vi "TicTacToev2.vi"() -> ()   [LabVIEW 2020]
panel:
  in  "Numeric":i32
  out "Who's Tern ?":bool
  out "Tank 2":i32(slide)
  out "players":dbl format="%#g"
  in  "LEVEL":i32(slide)=3000 scale=5.0..1.0
  out "Tank":i32(slide)
  out "Human(GREEN) Win":dbl
  out "Computer(RED)Win":dbl
  out "Tie":bool
  out "No one Won":bool
  out "Computer Won":bool
  out "Human Won":bool
  out "Turn":string
  out "XO array":string[][](array[string])
  in  "START GAME":bool
  in  "Boolean 9":bool
  in  "Boolean 8":bool
  in  "Boolean 7":bool
  in  "Boolean 6":bool
  in  "Boolean 5":bool
  in  "Boolean 4":bool
  in  "Boolean 3":bool
  in  "Boolean 2":bool
  in  "Boolean":bool
  in  "STOP GAME":bool
  in  "Turn":bool
  out "Game Over":bool
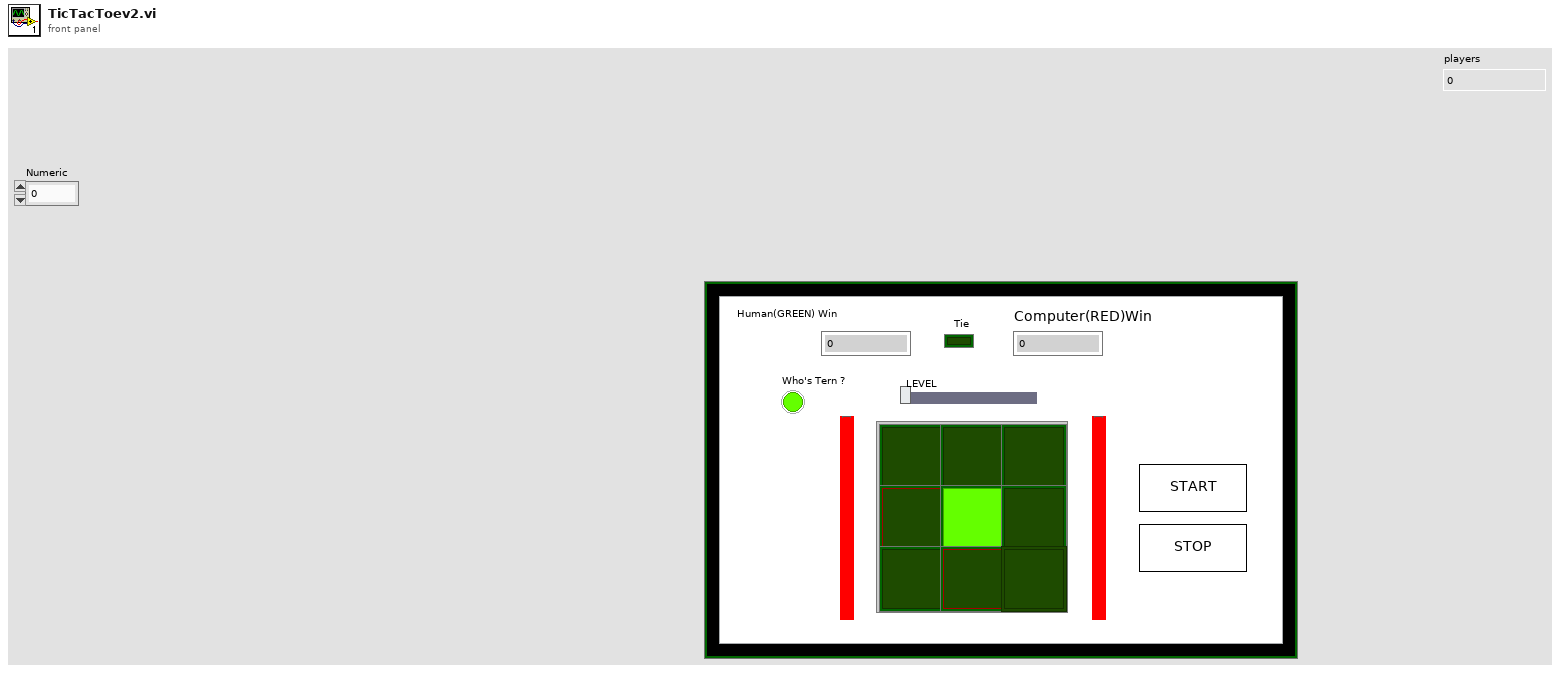
[diagram p1: front panel]
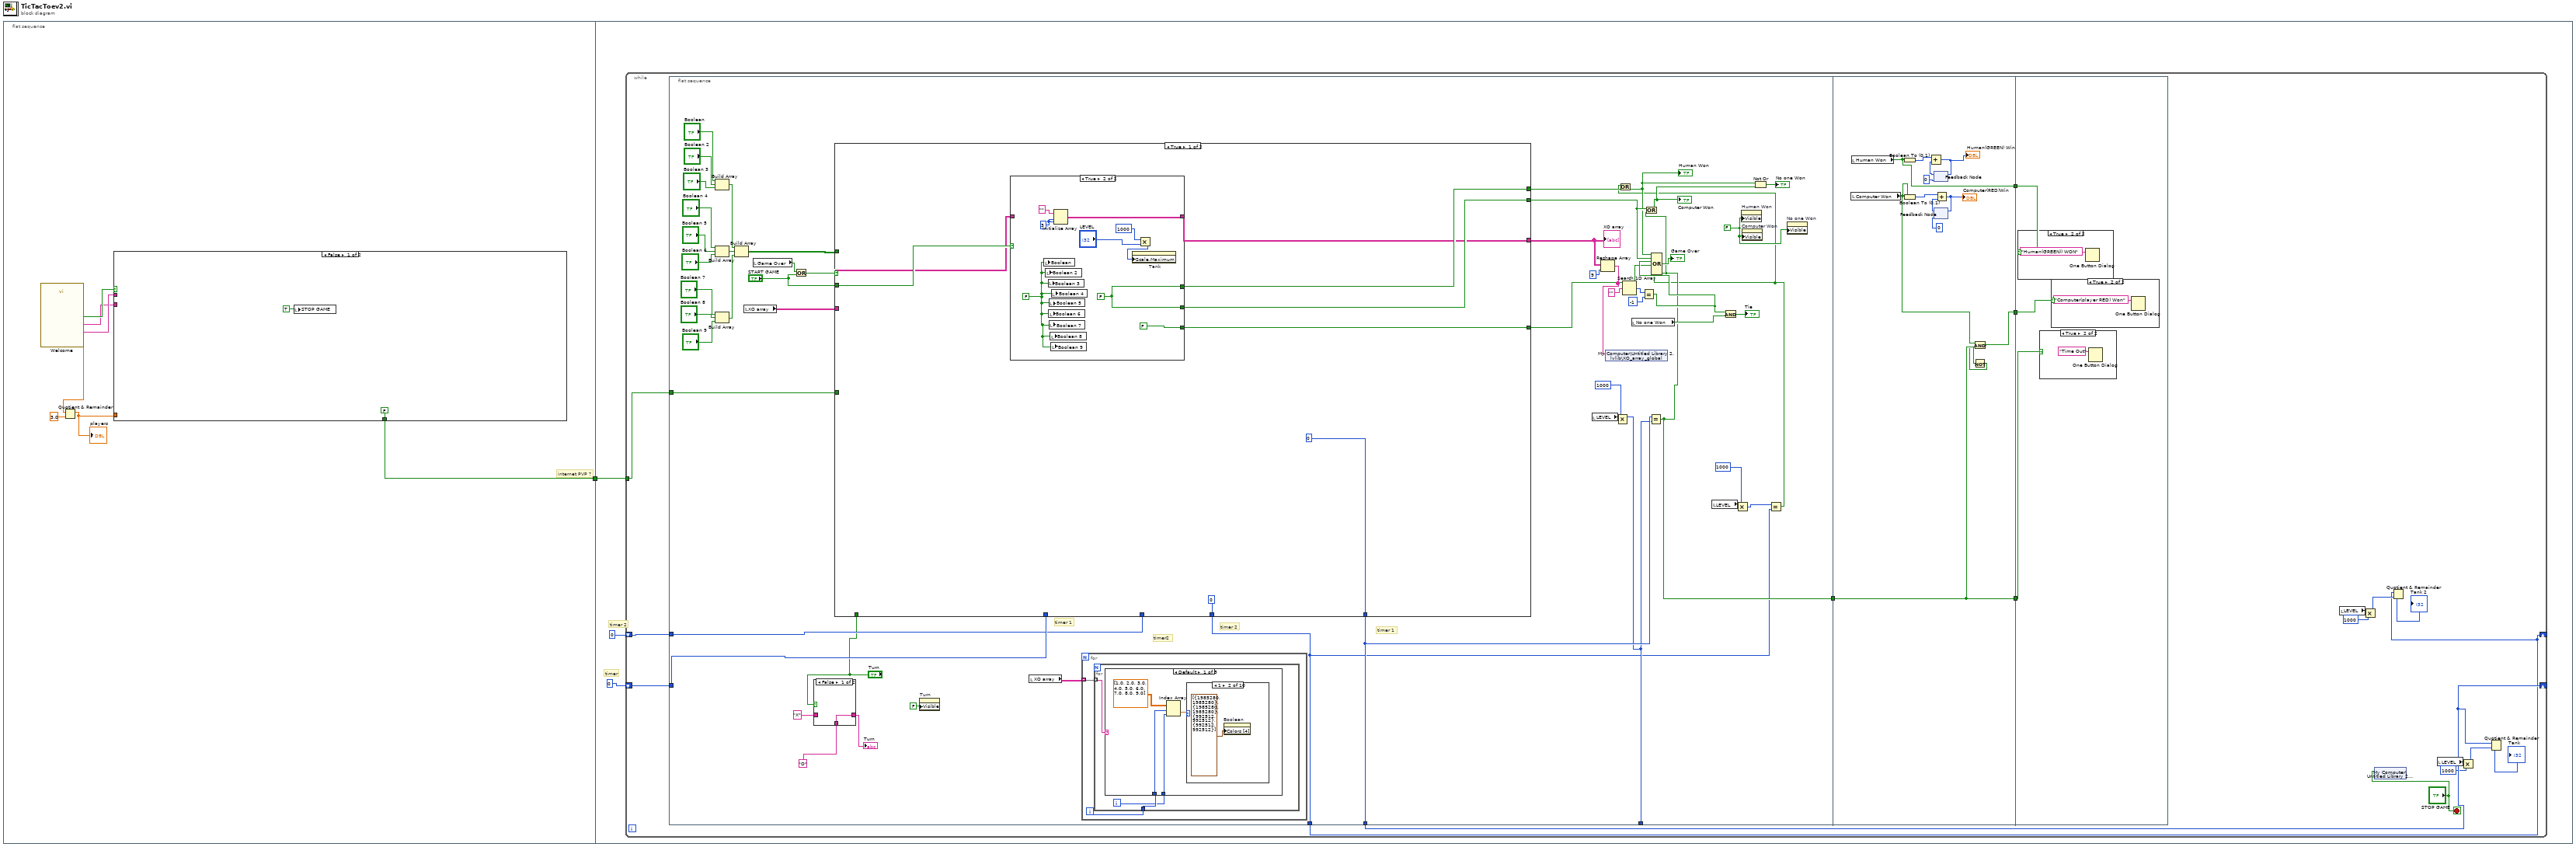
[diagram p0: block diagram]
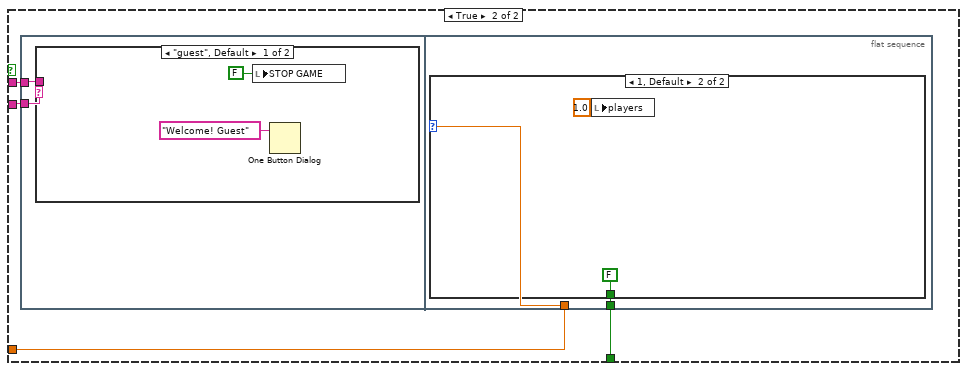
[diagram p2: hidden frame]
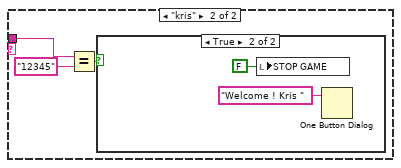
[diagram p3: hidden frame]
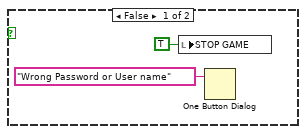
[diagram p4: hidden frame]
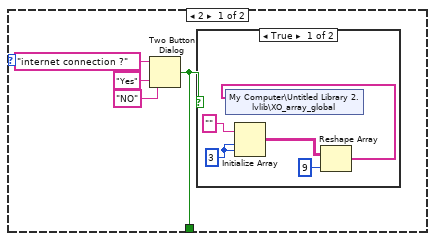
[diagram p5: hidden frame]
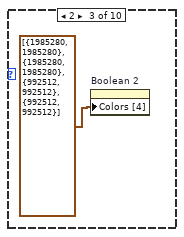
[diagram p8: hidden frame]
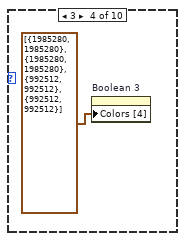
[diagram p9: hidden frame]
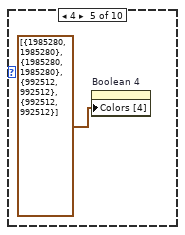
[diagram p10: hidden frame]
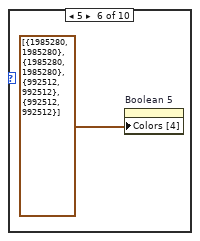
[diagram p11: hidden frame]
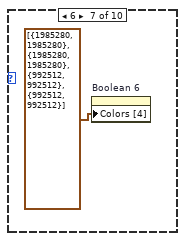
[diagram p12: hidden frame]
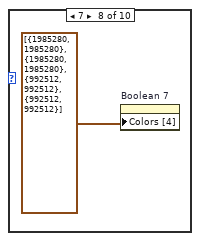
[diagram p13: hidden frame]
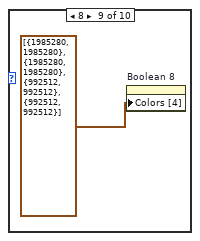
[diagram p14: hidden frame]
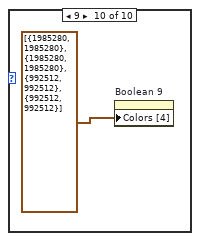
[diagram p15: hidden frame]
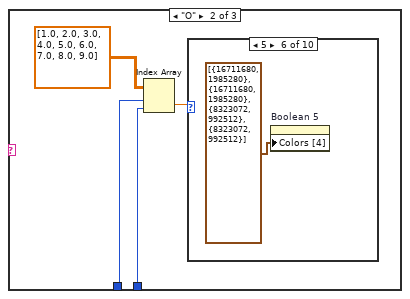
[diagram p16: hidden frame]
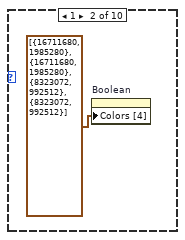
[diagram p18: hidden frame]
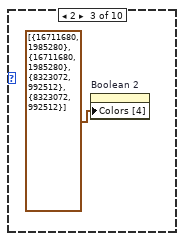
[diagram p19: hidden frame]
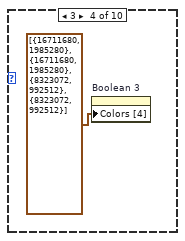
[diagram p20: hidden frame]
diagram:
  n1 = flat-sequence {
    tunnel: [w2] -> w1
    tunnel: w1 -> [w39]
    frame #0 {
      # "internet PVP ?"
      n2 = call "Welcome"() -> ("players(1 or 2 )"=w8:dbl, "password"=w5:string, "name"=w4:string, "OK"=w7:bool)  [unwired: 15 in, 1 out]
      n3 = Quotient & Remainder(x=w8, y=3.0) -> (x-y*floor(x/y)=w3:dbl)  [unwired: 1 out]
      "players" <- w3
      n4 = case shown="False" w7 {
        tunnel: w4 -> [_ w14]
        tunnel: w5 -> [_ w13]
        tunnel: w3 -> [_ w12]
        tunnel: [FALSE ("T button?") w11] -> w2
        frame False {
          n5 = local write "STOP GAME"(TRUE ("STOP GAME")) -> ()
        }
        frame True {
          n6 = flat-sequence {
            tunnel: w14 -> [w16]
            tunnel: w13 -> [w15]
            tunnel: w12 -> [w27]
            tunnel: [w26] -> w11
            frame #0 {
              n7 = case shown="\"guest\", Default" w16 {
                tunnel: w15 -> [_ w21]
                frame "guest", Default {
                  n8 = local write "STOP GAME"(FALSE ("STOP GAME")) -> ()
                  n9 = One Button Dialog(message="Welcome! Guest") -> ()  [unwired: 1 in, 1 out]
                }
                frame "kris" {
                  n10 = Equal?(x=w21, y="12345") -> (x = y?=w19:bool)
                  n11 = case shown="True" w19 {
                    frame False {
                      n12 = local write "STOP GAME"(TRUE ("STOP GAME")) -> ()
                      n13 = One Button Dialog(message="Wrong Password or User name") -> ()  [unwired: 1 in, 1 out]
                    }
                    frame True {
                      n14 = local write "STOP GAME"(FALSE ("STOP GAME")) -> ()
                      n15 = One Button Dialog(message="Welcome ! Kris ") -> ()  [unwired: 1 in, 1 out]
                    }
                  }
                }
              }
            }
            frame #1 {
              n16 = case shown="1, Default" w27 {
                tunnel: [w28 FALSE ("T button?")] -> w26
                frame 2 {
                  n17 = Two Button Dialog(message="internet connection ?", 1:"NO" ("F button name (\"Cancel\")"), 2:"Yes" ("T button name (\"OK\")")) -> (T button?=w28:bool)
                  n18 = case shown="True" w28 {
                    frame True {
                      w36 = 3
                      n19 = Initialize Array("", w36, w36) -> (w33:string[][])
                      n20 = Reshape Array(w33, 9 ("dimension size")) -> (w32:string[])
                      n21 = shared-variable "My Computer\\Untitled Library 2.lvlib\\XO_array_global"(w32) -> ()  [unwired: 1 in, 1 out]
                    }
                    frame False {
                    }
                  }
                }
                frame 1, Default {
                  n22 = local write "players"(1.0 ("players")) -> ()
                }
              }
            }
          }
        }
      }
    }
    frame #1 {
      # "timer 2"
      # "timer"
      n23 = while {
        shift-right: [w55] -> _
        shift-left: 0 -> [w57]
        shift-right: [w44] -> _
        shift-left: 0 -> [w49]
        tunnel: w39 -> [w42]
        stop <- "STOP GAME" stop-if-true
        n24 = flat-sequence {
          tunnel: [w75] -> w55
          tunnel: [w73] -> w53
          tunnel: [w71] -> _
          tunnel: w57 -> [w76]
          tunnel: w49 -> [w69]
          tunnel: [w65] -> w44
          tunnel: w42 -> [w61]
          tunnel: [w316] -> w59
          tunnel: [w319] -> w58
          tunnel: [w318] -> w54
          tunnel: w53 -> [w318]
          tunnel: w59 -> [w330]
          tunnel: w58 -> [w329]
          tunnel: w54 -> [w328]
          frame #0 {
            w78 = FALSE ("Visible")
            # "timer 1"
            # "timer 2"
            # "timer 1"
            # "timer2"
            n25 = Build Array("Boolean", "Boolean 2", "Boolean 3") -> (w110:bool[])
            n26 = Build Array("Boolean 4", "Boolean 5", "Boolean 6") -> (w111:bool[])
            n27 = Build Array("Boolean 7", "Boolean 8", "Boolean 9") -> (w112:bool[])
            n28 = Build Array(w110, w111, w112) -> (w102:bool[][])
            n29 = local read "XO array"() -> (w101:string[][])
            n30 = local read "Game Over"() -> (w94:bool)
            n31 = Or(x=w94, y="START GAME") -> (x .or. y?=w93:bool)
            n32 = case shown="False" "Turn" {
              tunnel: "X" -> [_ w158]
              tunnel: [w157 w158] -> w99
              tunnel: "O" ("x") -> [w157 _]
              frame False {
              }
              frame True {
              }
            }
            "Turn" <- w99
            n33 = case shown="True" w93 {
              tunnel: w102 -> [_ w200]
              tunnel: w101 -> [w165 w199]
              tunnel: "Turn" -> [_ w198]
              tunnel: "START GAME" -> [w166 _]
              tunnel: [w164 w191] -> w80
              tunnel: [w163 w190] -> w79
              tunnel: [w162 w189] -> w83
              tunnel: [w161 FALSE] -> w77
              tunnel: w76 -> [_ w187]
              tunnel: [0 w186] -> w75
              tunnel: w69 -> [_ w185]
              tunnel: [0 w184] -> w65
              tunnel: w61 -> [_ w180]
              frame True {
                n34 = case shown="True" w166 {
                  tunnel: [w169 w177] -> w162
                  tunnel: [w168 w176] -> w163
                  tunnel: [w168 w176] -> w164
                  tunnel: w165 -> [w169 _]
                  tunnel: [TRUE FALSE] -> w161
                  frame False {
                    w168 = FALSE
                  }
                  frame True {
                    w174 = FALSE
                    w176 = FALSE
                    w175 = 3
                    n35 = local write "Boolean"(w174) -> ()
                    n36 = local write "Boolean 2"(w174) -> ()
                    n37 = local write "Boolean 3"(w174) -> ()
                    n38 = local write "Boolean 6"(w174) -> ()
                    n39 = local write "Boolean 5"(w174) -> ()
                    n40 = local write "Boolean 7"(w174) -> ()
                    n41 = local write "Boolean 8"(w174) -> ()
                    n42 = local write "Boolean 9"(w174) -> ()
                    n43 = local write "Boolean 4"(w174) -> ()
                    n44 = Initialize Array("", w175, w175) -> (w177:string[][])
                    n45 = Multiply(x=1000, y="LEVEL") -> (x*y=w170:i32)
                    n46 = property on="Tank" class="Slide (strict)"("Scale.Maximum"=w170) -> ()  [unwired: 2 in, 2 out]
                  }
                }
              }
              frame False {
                n47 = local read "Turn"() -> (w179:string)
                n48 = shared-variable "My Computer\\Untitled Library 2.lvlib\\Turn_string"(w179) -> ()  [unwired: 1 in, 1 out]
                n49 = Equal?(x=w179, y="O") -> (x = y?=w182:bool)
                n50 = case shown="False" w182 {
                  frame False {
                    n51 = property on="Who's Tern ?" class="Bool (strict)"("Colors [4]"=cluster{u32, u32}[] [{6618880, 6618880}]) -> ()  [unwired: 2 in, 2 out]
                  }
                  frame True {
                    n52 = property on="Who's Tern ?" class="Bool (strict)"("Colors [4]"=cluster{u32, u32}[] [{16711680, 16711680}]) -> ()  [unwired: 2 in, 2 out]
                  }
                }
                n53 = case shown="False" w198 {
                  tunnel: w200 -> [w213 w285]
                  tunnel: w199 -> [w215 w284]
                  tunnel: [w216 w283] -> w189
                  tunnel: w179 -> [w212 w282]
                  tunnel: w187 -> [w208 w280]
                  tunnel: [w211 w279] -> w186
                  tunnel: w185 -> [w210 _]
                  tunnel: [w209 0] -> w184
                  tunnel: w180 -> [w207 _]
                  frame False {
                    n54 = local read "players"() -> (w214:dbl)
                    n55 = case shown="2" w214 {
                      tunnel: [w221 w276] -> w216
                      tunnel: w215 -> [w224 w275]
                      tunnel: w213 -> [w222 _]
                      tunnel: w212 -> [w223 _]
                      tunnel: w210 -> [w220 _]
                      tunnel: [0 0] -> w211
                      tunnel: [w219 0] -> w209
                      tunnel: w208 -> [_ _]
                      tunnel: w207 -> [w217 _]
                      frame 2 {
                        # "connect to timer2"
                        n56 = case shown="True" w217 {
                          tunnel: w224 -> [_ w240]
                          tunnel: w223 -> [_ w239]
                          tunnel: w222 -> [_ w238]
                          tunnel: [w226 w237] -> w221
                          tunnel: w220 -> [_ w236]
                          tunnel: ["Numeric" w235] -> w219
                          frame True {
                            n57 = flat-sequence {
                              tunnel: [w233] -> w226
                              frame #0 {
                                n58 = while {
                                stop <- w229 stop-if-true
                                n59 = shared-variable "My Computer\\Untitled Library 2.lvlib\\Internet_PVP"(TRUE ("Internet_PVP")) -> ()  [unwired: 1 in, 1 out]
                                n60 = shared-variable "My Computer\\Untitled Library 2.lvlib\\Turn"(FALSE ("Turn")) -> ()  [unwired: 1 in, 1 out]
                                n61 = shared-variable "My Computer\\Untitled Library 2.lvlib\\Client_end"() -> (w229:bool)  [unwired: 1 in, 1 out]
                                n62 = shared-variable "My Computer\\Untitled Library 2.lvlib\\timer_2"() -> (w228:i32)  [unwired: 1 in, 1 out]
                                n63 = local write "Numeric"(w228) -> ()
                                }
                              }
                              frame #1 {
                                n64 = shared-variable "My Computer\\Untitled Library 2.lvlib\\XO_array_global"() -> (w234:string[])  [unwired: 1 in, 1 out]
                                n65 = Reshape Array(w234, 3 ("dimension size"), 3 ("dimension size")) -> (w233:string[][])
                              }
                            }
                          }
                          frame False {
                            w241 = 3
                            n66 = for {
                              N: w241 -> [_]
                              tunnel: w241 -> [w248]
                              tunnel: w238 -> [w247] mode=indexing
                              tunnel: w240 -> [w246] mode=indexing
                              tunnel: [w245] -> w237 mode=indexing
                              tunnel: w239 -> [w244]
                              tunnel: w236 -> [w243]
                              tunnel: [w242] -> w235
                              n67 = for {
                                N: w248 -> [_]
                                tunnel: w247 -> [w258] mode=indexing
                                tunnel: w246 -> [w255] mode=indexing
                                tunnel: w244 -> [w253]
                                tunnel: [w254] -> w245 mode=indexing
                                tunnel: w243 -> [w250]
                                tunnel: [w249] -> w242
                                n68 = Not Equal?(x=w255, y="X") -> (x != y?=w259:bool)
                                n69 = Not Equal?(x="O", y=w255) -> (x != y?=w260:bool)
                                n70 = And(x=w260, y=w259) -> (x .and. y?=w257:bool)
                                n71 = local read "Turn"() -> (w252:bool)
                                n72 = And(x=w258, y=w257) -> (x .and. y?=w256:bool)
                                n73 = case shown="True" w256 {
                                tunnel: w255 -> [w266 _]
                                tunnel: [w266 w268] -> w254
                                tunnel: w253 -> [_ w268]
                                tunnel: [w265 w269] -> w251
                                tunnel: w252 -> [w265 w270]
                                tunnel: w250 -> [w264 _]
                                tunnel: [w263 0] -> w249
                                frame False {
                                n74 = Increment(x=w264) -> (x+1=w263:i32)
                                }
                                frame True {
                                n75 = Not(x=w270) -> (.not. x?=w269:bool)
                                }
                                }
                                n76 = local write "Turn"(w251) -> ()
                              }
                            }
                          }
                        }
                      }
                      frame 1, Default {
                        n77 = local read "Turn"() -> (w274:bool)
                        n78 = call "AI algorithm(SubVI).vi"("Turn"=w274, "XO array"=w275) -> ("Turn 2"=w273:bool, "XO array 2"=w276:string[][])
                        n79 = local write "Turn"(w273) -> ()
                      }
                    }
                  }
                  frame True {
                    w281 = 3
                    n80 = for {
                      N: w281 -> [_]
                      tunnel: w281 -> [w292]
                      tunnel: w285 -> [w291] mode=indexing
                      tunnel: w284 -> [w290] mode=indexing
                      tunnel: [w289] -> w283 mode=indexing
                      tunnel: w282 -> [w288]
                      tunnel: w280 -> [w287]
                      tunnel: [w286] -> w279
                      n81 = for {
                        N: w292 -> [_]
                        tunnel: w291 -> [w302] mode=indexing
                        tunnel: w290 -> [w300] mode=indexing
                        tunnel: w288 -> [w298]
                        tunnel: [w299] -> w289 mode=indexing
                        tunnel: w287 -> [w294]
                        tunnel: [w293] -> w286
                        n82 = Not Equal?(x=w300, y="X") -> (x != y?=w303:bool)
                        n83 = Not Equal?(x="O", y=w300) -> (x != y?=w304:bool)
                        n84 = And(x=w304, y=w303) -> (x .and. y?=w301:bool)
                        n85 = local read "Turn"() -> (w296:bool)
                        n86 = And(x=w302, y=w301) -> (x .and. y?=w295:bool)
                        n87 = case shown="True" w295 {
                          tunnel: w300 -> [w310 _]
                          tunnel: [w310 w312] -> w299
                          tunnel: w298 -> [_ w312]
                          tunnel: [w309 w313] -> w297
                          tunnel: w296 -> [w309 w314]
                          tunnel: w294 -> [w308 _]
                          tunnel: [w307 0] -> w293
                          frame False {
                            n88 = Increment(x=w308) -> (x+1=w307:i32)
                          }
                          frame True {
                            n89 = Not(x=w314) -> (.not. x?=w313:bool)
                          }
                        }
                        n90 = local write "Turn"(w297) -> ()
                      }
                    }
                    n91 = shared-variable "My Computer\\Untitled Library 2.lvlib\\timer_2"(0 ("timer_2")) -> ()  [unwired: 1 in, 1 out]
                  }
                }
                n92 = call "CheckWinDiag(SubVI).vi"("Array"=w189) -> ("x .or. y?"=w196:bool)  [unwired: 10 in]
                n93 = Transpose 2D Array(2D array=w189) -> (transposed array=w197:string[][])
                n94 = call "CheckWinRow(SubVI).vi"("Array"=w189) -> ("x .or. y? 2"=w195:bool)  [unwired: 10 in]
                n95 = call "CheckWinRow(SubVI).vi"("Array"=w197) -> ("x .or. y? 2"=w194:bool)  [unwired: 10 in]
                n96 = local read "Turn"() -> (w192:string)
                n97 = Compound Arithmetic op=OR(w196, w195, w194) -> (w193:bool)
                n98 = case shown="\"O\", Default" w192 {
                  tunnel: w193 -> [w204 w205]
                  tunnel: [w204 FALSE] -> w191
                  tunnel: [FALSE w205] -> w190
                  frame "O", Default {
                  }
                  frame "X" {
                  }
                }
                "Who's Tern ?" <- TRUE ("Boolean 10")
              }
            }
            "XO array" <- w83
            n99 = property on="Turn" class="Bool (strict)"("Visible"=FALSE) -> ()  [unwired: 2 in, 2 out]
            n100 = local read "XO array"() -> (w82:string[][])
            n101 = for {
              tunnel: w82 -> [w113] mode=indexing
              i -> [w114]
              n102 = for {
                tunnel: w114 -> [w117]
                tunnel: w113 -> [w115] mode=indexing
                i -> [w116]
                n103 = case shown="Default" w115 {
                  tunnel: w117 -> [w121 w132 w145]
                  tunnel: w116 -> [w120 w131 w146]
                  frame Default {
                    n104 = Index Array(array=dbl[][] [[1.0, 2.0, 3.0], [4.0, 5.0, 6.0], [7.0, 8.0, 9.0]] ("Array"), index (row)=w121, index (col)=w120) -> (element=w118:dbl)
                    n105 = case shown="1" w118 {
                      frame 0, Default {
                      }
                      frame 1 {
                        n106 = property on="Boolean" class="Bool (strict)"("Colors [4]"=cluster{u32, u32}[] [{1985280, 1985280}, {1985280, 1985280}, {992512, 992512}, {992512, 992512}]) -> ()  [unwired: 2 in, 2 out]
                      }
                      frame 2 {
                        n107 = property on="Boolean 2" class="Bool (strict)"("Colors [4]"=cluster{u32, u32}[] [{1985280, 1985280}, {1985280, 1985280}, {992512, 992512}, {992512, 992512}]) -> ()  [unwired: 2 in, 2 out]
                      }
                      frame 3 {
                        n108 = property on="Boolean 3" class="Bool (strict)"("Colors [4]"=cluster{u32, u32}[] [{1985280, 1985280}, {1985280, 1985280}, {992512, 992512}, {992512, 992512}]) -> ()  [unwired: 2 in, 2 out]
                      }
                      frame 4 {
                        n109 = property on="Boolean 4" class="Bool (strict)"("Colors [4]"=cluster{u32, u32}[] [{1985280, 1985280}, {1985280, 1985280}, {992512, 992512}, {992512, 992512}]) -> ()  [unwired: 2 in, 2 out]
                      }
                      frame 5 {
                        n110 = property on="Boolean 5" class="Bool (strict)"("Colors [4]"=cluster{u32, u32}[] [{1985280, 1985280}, {1985280, 1985280}, {992512, 992512}, {992512, 992512}]) -> ()  [unwired: 2 in, 2 out]
                      }
                      frame 6 {
                        n111 = property on="Boolean 6" class="Bool (strict)"("Colors [4]"=cluster{u32, u32}[] [{1985280, 1985280}, {1985280, 1985280}, {992512, 992512}, {992512, 992512}]) -> ()  [unwired: 2 in, 2 out]
                      }
                      frame 7 {
                        n112 = property on="Boolean 7" class="Bool (strict)"("Colors [4]"=cluster{u32, u32}[] [{1985280, 1985280}, {1985280, 1985280}, {992512, 992512}, {992512, 992512}]) -> ()  [unwired: 2 in, 2 out]
                      }
                      frame 8 {
                        n113 = property on="Boolean 8" class="Bool (strict)"("Colors [4]"=cluster{u32, u32}[] [{1985280, 1985280}, {1985280, 1985280}, {992512, 992512}, {992512, 992512}]) -> ()  [unwired: 2 in, 2 out]
                      }
                      frame 9 {
                        n114 = property on="Boolean 9" class="Bool (strict)"("Colors [4]"=cluster{u32, u32}[] [{1985280, 1985280}, {1985280, 1985280}, {992512, 992512}, {992512, 992512}]) -> ()  [unwired: 2 in, 2 out]
                      }
                    }
                  }
                  frame "O" {
                    n115 = Index Array(array=dbl[][] [[1.0, 2.0, 3.0], [4.0, 5.0, 6.0], [7.0, 8.0, 9.0]] ("Array"), index (row)=w132, index (col)=w131) -> (element=w133:dbl)
                    n116 = case shown="5" w133 {
                      frame 0, Default {
                      }
                      frame 1 {
                        n117 = property on="Boolean" class="Bool (strict)"("Colors [4]"=cluster{u32, u32}[] [{16711680, 1985280}, {16711680, 1985280}, {8323072, 992512}, {8323072, 992512}]) -> ()  [unwired: 2 in, 2 out]
                      }
                      frame 2 {
                        n118 = property on="Boolean 2" class="Bool (strict)"("Colors [4]"=cluster{u32, u32}[] [{16711680, 1985280}, {16711680, 1985280}, {8323072, 992512}, {8323072, 992512}]) -> ()  [unwired: 2 in, 2 out]
                      }
                      frame 3 {
                        n119 = property on="Boolean 3" class="Bool (strict)"("Colors [4]"=cluster{u32, u32}[] [{16711680, 1985280}, {16711680, 1985280}, {8323072, 992512}, {8323072, 992512}]) -> ()  [unwired: 2 in, 2 out]
                      }
                      frame 4 {
                        n120 = property on="Boolean 4" class="Bool (strict)"("Colors [4]"=cluster{u32, u32}[] [{16711680, 1985280}, {16711680, 1985280}, {8323072, 992512}, {8323072, 992512}]) -> ()  [unwired: 2 in, 2 out]
                      }
                      frame 5 {
                        n121 = property on="Boolean 5" class="Bool (strict)"("Colors [4]"=cluster{u32, u32}[] [{16711680, 1985280}, {16711680, 1985280}, {8323072, 992512}, {8323072, 992512}]) -> ()  [unwired: 2 in, 2 out]
                      }
                      frame 6 {
                        n122 = property on="Boolean 6" class="Bool (strict)"("Colors [4]"=cluster{u32, u32}[] [{16711680, 1985280}, {16711680, 1985280}, {8323072, 992512}, {8323072, 992512}]) -> ()  [unwired: 2 in, 2 out]
                      }
                      frame 7 {
                        n123 = property on="Boolean 7" class="Bool (strict)"("Colors [4]"=cluster{u32, u32}[] [{16711680, 1985280}, {16711680, 1985280}, {8323072, 992512}, {8323072, 992512}]) -> ()  [unwired: 2 in, 2 out]
                      }
                      frame 8 {
                        n124 = property on="Boolean 8" class="Bool (strict)"("Colors [4]"=cluster{u32, u32}[] [{16711680, 1985280}, {16711680, 1985280}, {8323072, 992512}, {8323072, 992512}]) -> ()  [unwired: 2 in, 2 out]
                      }
                      frame 9 {
                        n125 = property on="Boolean 9" class="Bool (strict)"("Colors [4]"=cluster{u32, u32}[] [{16711680, 1985280}, {16711680, 1985280}, {8323072, 992512}, {8323072, 992512}]) -> ()  [unwired: 2 in, 2 out]
                      }
                    }
                  }
                  frame "X" {
                    n126 = Index Array(array=dbl[][] [[1.0, 2.0, 3.0], [4.0, 5.0, 6.0], [7.0, 8.0, 9.0]] ("Array"), index (row)=w145, index (col)=w146) -> (element=w147:dbl)
                    n127 = case shown="1" w147 {
                      frame 0, Default {
                      }
                      frame 1 {
                        n128 = property on="Boolean" class="Bool (strict)"("Colors [4]"=cluster{u32, u32}[] [{6618880, 6618880}, {6618880, 6618880}, {3309312, 3309312}, {3309312, 3309312}]) -> ()  [unwired: 2 in, 2 out]
                      }
                      frame 2 {
                        n129 = property on="Boolean 2" class="Bool (strict)"("Colors [4]"=cluster{u32, u32}[] [{6618880, 6618880}, {6618880, 6618880}, {3309312, 3309312}, {3309312, 3309312}]) -> ()  [unwired: 2 in, 2 out]
                      }
                      frame 3 {
                        n130 = property on="Boolean 3" class="Bool (strict)"("Colors [4]"=cluster{u32, u32}[] [{6618880, 6618880}, {6618880, 6618880}, {3309312, 3309312}, {3309312, 3309312}]) -> ()  [unwired: 2 in, 2 out]
                      }
                      frame 4 {
                        n131 = property on="Boolean 4" class="Bool (strict)"("Colors [4]"=cluster{u32, u32}[] [{6618880, 6618880}, {6618880, 6618880}, {3309312, 3309312}, {3309312, 3309312}]) -> ()  [unwired: 2 in, 2 out]
                      }
                      frame 5 {
                        n132 = property on="Boolean 5" class="Bool (strict)"("Colors [4]"=cluster{u32, u32}[] [{6618880, 6618880}, {6618880, 6618880}, {3309312, 3309312}, {3309312, 3309312}]) -> ()  [unwired: 2 in, 2 out]
                      }
                      frame 6 {
                        n133 = property on="Boolean 6" class="Bool (strict)"("Colors [4]"=cluster{u32, u32}[] [{6618880, 6618880}, {6618880, 6618880}, {3309312, 3309312}, {3309312, 3309312}]) -> ()  [unwired: 2 in, 2 out]
                      }
                      frame 7 {
                        n134 = property on="Boolean 7" class="Bool (strict)"("Colors [4]"=cluster{u32, u32}[] [{6618880, 6618880}, {6618880, 6618880}, {3309312, 3309312}, {3309312, 3309312}]) -> ()  [unwired: 2 in, 2 out]
                      }
                      frame 8 {
                        n135 = property on="Boolean 8" class="Bool (strict)"("Colors [4]"=cluster{u32, u32}[] [{6618880, 6618880}, {6618880, 6618880}, {3309312, 3309312}, {3309312, 3309312}]) -> ()  [unwired: 2 in, 2 out]
                      }
                      frame 9 {
                        n136 = property on="Boolean 9" class="Bool (strict)"("Colors [4]"=cluster{u32, u32}[] [{6618880, 6618880}, {6618880, 6618880}, {3309312, 3309312}, {3309312, 3309312}]) -> ()  [unwired: 2 in, 2 out]
                      }
                    }
                  }
                }
              }
            }
            n137 = local read "LEVEL"() -> (w72:i32)
            n138 = Reshape Array(w83, 9 ("dimension size")) -> (w62:string[])
            n139 = shared-variable "My Computer\\Untitled Library 2.lvlib\\XO_array_global"(w62) -> ()  [unwired: 1 in, 1 out]
            n140 = Multiply(x=w72, y=1000) -> (x*y=w71:i32)
            n141 = Search 1D Array(1D array=w62, element="") -> (index of element=w87:i32)  [unwired: 1 in]
            n142 = local read "No one Won"() -> (w90:bool)
            n143 = Equal?(x=w87, y=-1) -> (x = y?=w84:bool)
            n144 = Equal?(x=w75, y=w71) -> (x = y?=w73:bool)
            n145 = Or(x=w80, y=w73) -> (x .or. y?=w74:bool)
            "Computer Won" <- w74
            n146 = local read "LEVEL"() -> (w67:i32)
            n147 = And(x=w84, y=w90) -> (x .and. y?=→"Tie":bool)
            n148 = Multiply(x=w67, y=1000) -> (x*y=w66:i32)
            n149 = property on="Human Won" class="Bool (strict)"("Visible"=w78) -> ()  [unwired: 2 in, 2 out]
            n150 = property on="Computer Won" class="Bool (strict)"("Visible"=w78) -> ()  [unwired: 2 in, 2 out]
            n151 = Equal?(x=w66, y=w65) -> (x = y?=w63:bool)
            n152 = Or(x=w63, y=w79) -> (x .or. y?=w64:bool)
            "Human Won" <- w64
            n153 = Compound Arithmetic op=OR(w64, w80, w84, w77, w73, w63) -> (→"Game Over":bool)
            n154 = Not Or(1:w74, 2:w64) -> (0:→"No one Won":bool)
            n155 = property on="No one Won" class="Bool (strict)"("Visible"=w78) -> ()  [unwired: 2 in, 2 out]
          }
          frame #1 {
            n156 = local read "Computer Won"() -> (w317:bool)
            n157 = local read "Human Won"() -> (w319:bool)
            n158 = Boolean To (0,1)(Boolean=w319) -> (0, 1=w322:i16)
            n159 = Boolean To (0,1)(Boolean=w317) -> (0, 1=w320:i16)
            n160 = feedback #1(i16 0) -> (w323:i16)
            n161 = Add(x=w322, y=w323) -> (x+y=w325:i16)
            "Human(GREEN) Win" <- w325
            n162 = feedback-in #1(w325) -> ()
            n163 = feedback #2(i16 0) -> (w321:i16)
            n164 = Add(x=w320, y=w321) -> (x+y=w324:i16)
            "Computer(RED)Win" <- w324
            n165 = feedback-in #2(w324) -> ()
            n166 = Not(x=w318) -> (.not. x?=w315:bool)
            n167 = And(x=w317, y=w315) -> (x .and. y?=w316:bool)
          }
          frame #2 {
            n168 = case shown="True" w329 {
              frame False {
              }
              frame True {
                n169 = One Button Dialog(message="Human(GREEN)) WON") -> ()  [unwired: 1 in, 1 out]
              }
            }
            n170 = case shown="True" w328 {
              frame False {
              }
              frame True {
                n171 = One Button Dialog(message="Time Out") -> ()  [unwired: 1 in, 1 out]
              }
            }
            n172 = case shown="True" w330 {
              frame False {
              }
              frame True {
                n173 = One Button Dialog(message="Computer(player RED) Won") -> ()  [unwired: 1 in, 1 out]
              }
            }
          }
        }
        n174 = local read "LEVEL"() -> (w46:i32)
        n175 = Multiply(x=w46, y=1000) -> (x*y=w47:i32)
        n176 = shared-variable "My Computer\\Untitled Library 2.lvlib\\stop"("STOP GAME") -> ()  [unwired: 1 in, 1 out]
        n177 = Quotient & Remainder(x=w44, y=w47) -> (x-y*floor(x/y)=→"Tank 2":i32)  [unwired: 1 out]
        n178 = local read "LEVEL"() -> (w52:i32)
        n179 = Multiply(x=w52, y=1000) -> (x*y=w51:i32)
        n180 = Quotient & Remainder(x=w55, y=w51) -> (x-y*floor(x/y)=→"Tank":i32)  [unwired: 1 out]
      }
    }
  }
